vi "Main_E727_MultichannelMove.vi"() -> ()   [LabVIEW 2022 SP3]
doc: "This VI demonstrates how to initialize an E-727 system, how to move one connected axis and how to query for the position value of this axis. \nIn this example the E-727 is connected through COM port 1 with baudrate 115200. The VI runs E727_Configuration_Setup.vi with these specified settings, moves the first connected axis relative to its current position and reads the position of this axis. The diagram shows how to combine the driver VIs for these tasks. \nWarning: Before running this VI, modify the \"Interface\" and \"RS232 settings\" (or TCP/IP settings or USB settings ) to reflect your configuration. The predefined settings provided with the VI probably do not match your system."
uses:
  C:/Users/101d/Documents/Princeton Instruments/LightField/Add-in and Automation SDK/Samples/LabVIEW Automation/lightfield-automation-labview/LightField Automation.lvclass
panel:
  in  "Experiment Name:":u16(ring) items=["600IRWide", "1200SiWide"]
  in  "Tab Control":enum32{"Referenced Move", "Non referenced move"}(tab)
  in  "Set Point 1":bool
  out "Point 1":dbl[](array[numeric])=[137.9507141, 145.0551147, 152.0245361] format="%.6f"
  out "Point 2":dbl[](array[numeric])=[138.5597992, 116.5416107, 151.9612579] format="%.6f"
  in  "Set Point 2":bool
  in  "Start Mapping":bool
  out "Starting location":dbl[](array[numeric])=[136.47789, 224.1664276, 151.9103088] format="%.6f"
  in  "Set Starting location":bool
  in  "Left(-)/Right(+)":bool=TRUE
  in  "Up(-)/Down(+)":bool=TRUE
  in  "Move to Point 1":bool
  in  "Move to Point 2":bool
  in  "Move to \nStarting location":bool
  out "Y Move history":dbl[](array[numeric])
  out "X Move history":dbl[](array[numeric])
  out "Corrected angle":dbl
  out "Abs y":dbl
  out "Abs x":dbl
  out "y point":dbl
  out "x point":dbl
  in  "Array distance, D (um)":dbl=28.51
  in  "Pitch (um)":dbl=4.8
  in  "NxN array size":i32
  out "Inital position":dbl[](array[numeric]) format="%.6f"
  in  "Relative Resolution (um)":dbl[](array[numeric]) format="%.6f"
  in  "Map size":i32=7
  in  "Type of Motion":bool=TRUE
  in  "Target AbsolutePosition (um)":dbl[](array[numeric])=[150.0, 150.0, 150.0] format="%.6f"
  out "StageRunning 2":bool
  out "StageRunning 3":bool
  in  "Start Move":bool
  in  "Shut down":bool
  out "Position":dbl[](array[numeric]) format="%.6f"
  out "StageChannels":string[](array[string])
  in  "X / Y Resolution (um)":dbl=1.0 min=1.0
  in  "Z Resolution (um)":dbl=1.0 min=1.0
  in  "Left x0.5":bool
  in  "Right x0.5":bool
  in  "Up x0.5":bool
  in  "Down x0.5":bool
  in  "Down Z x4":bool
  in  "Down Z x2":bool
  in  "Up Z x4":bool
  in  "Up Z x2":bool
  in  "Up Z":bool
  in  "Down Z":bool
  in  "Right x4":bool
  in  "Right x2":bool
  in  "Left x4":bool
  in  "Left x2":bool
  in  "Down x4":bool
  in  "Down x2":bool
  in  "Up x4":bool
  in  "Up x2":bool
  in  "Right":bool
  in  "Left":bool
  in  "Up":bool
  in  "Down":bool
  out "LFRunning":bool
  out "LFObject":refnum<class "LightField Automation.lvclass">
  in  "LightFieldOn/Off":bool
  out "Progress":dbl(slide) scale=0.0..100.0
  out "Loop counter":dbl
  in  "error in":errorcluster
  out "StageRunning":bool
  in  "StageOn/Off":bool
  out "Pre-move position":dbl[](array[numeric]) format="%.6f"
  in  "stop":bool
  out "error out":errorcluster
  out "Current position":dbl[](array[numeric]) format="%.6f"
  # "Free relative move"
  # "Z Focus"
  # "X / Y Navigation"
  # "Lightfield"
  # "Y\nX\nZ"
  # "Flick to the direction of scan you want.\ne.g. default will move mapping right and up.\ngoing from bottom left to top right"
  # "Relative mapping\nRequires lightfield to be \"on\"\nThis will perform scans based on relative position and move in an \"S\" shape\nRelative solution is the length the stage will move per scan both in the X and Y axis\nMap size is the NxN scans it will take"
  # "Relative motion"
  # "Absolute motion"
  # "Relative Mapping settings"
  # "Y"
  # "X"
  # "Relative moving path"
  # "Z"
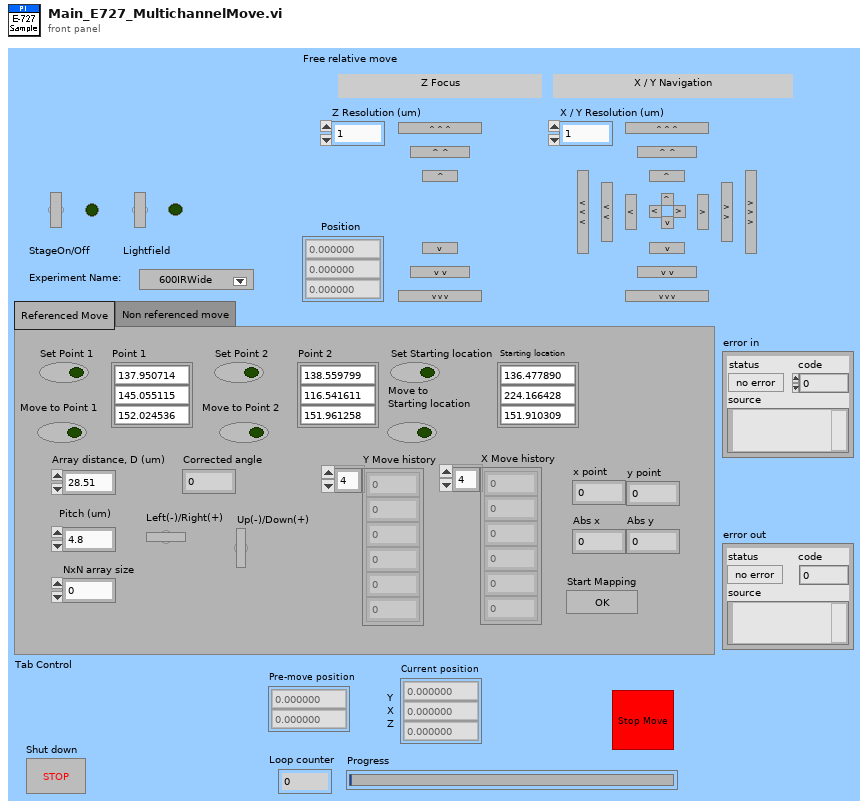
[diagram p1: front panel]
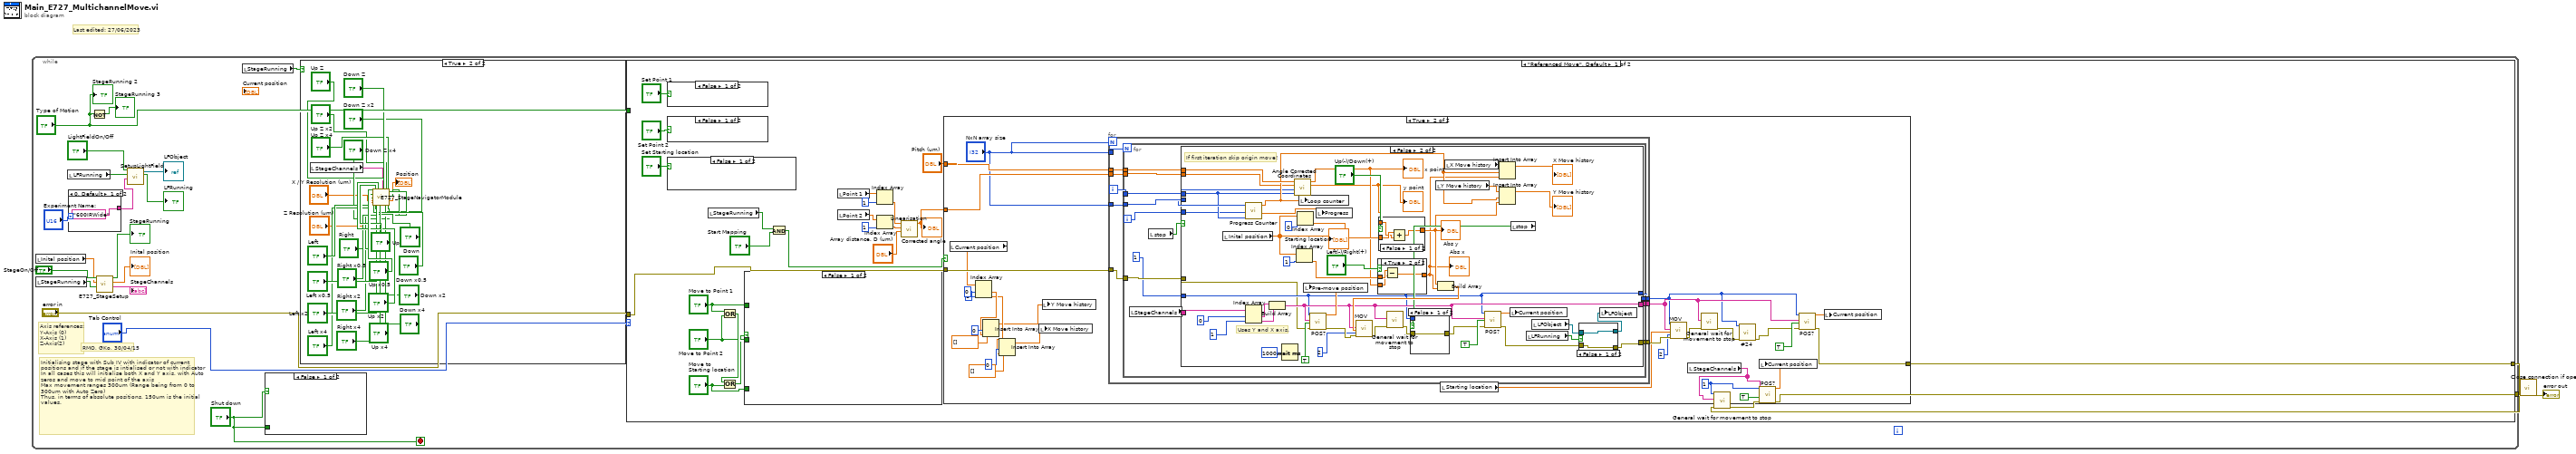
[diagram p0: block diagram]
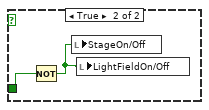
[diagram p2: hidden frame]
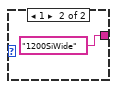
[diagram p3: hidden frame]
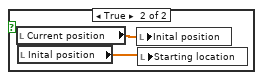
[diagram p4: hidden frame]
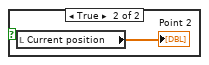
[diagram p5: hidden frame]
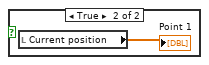
[diagram p6: hidden frame]
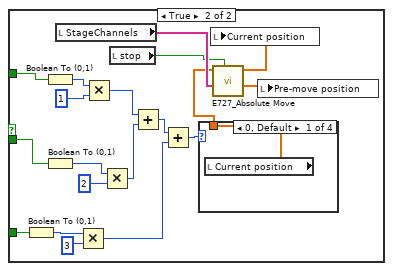
[diagram p7: hidden frame]
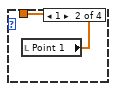
[diagram p8: hidden frame]
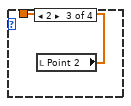
[diagram p9: hidden frame]
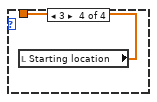
[diagram p10: hidden frame]
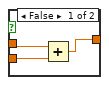
[diagram p13: hidden frame]
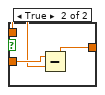
[diagram p14: hidden frame]
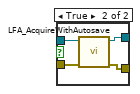
[diagram p15: hidden frame]
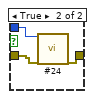
[diagram p16: hidden frame]
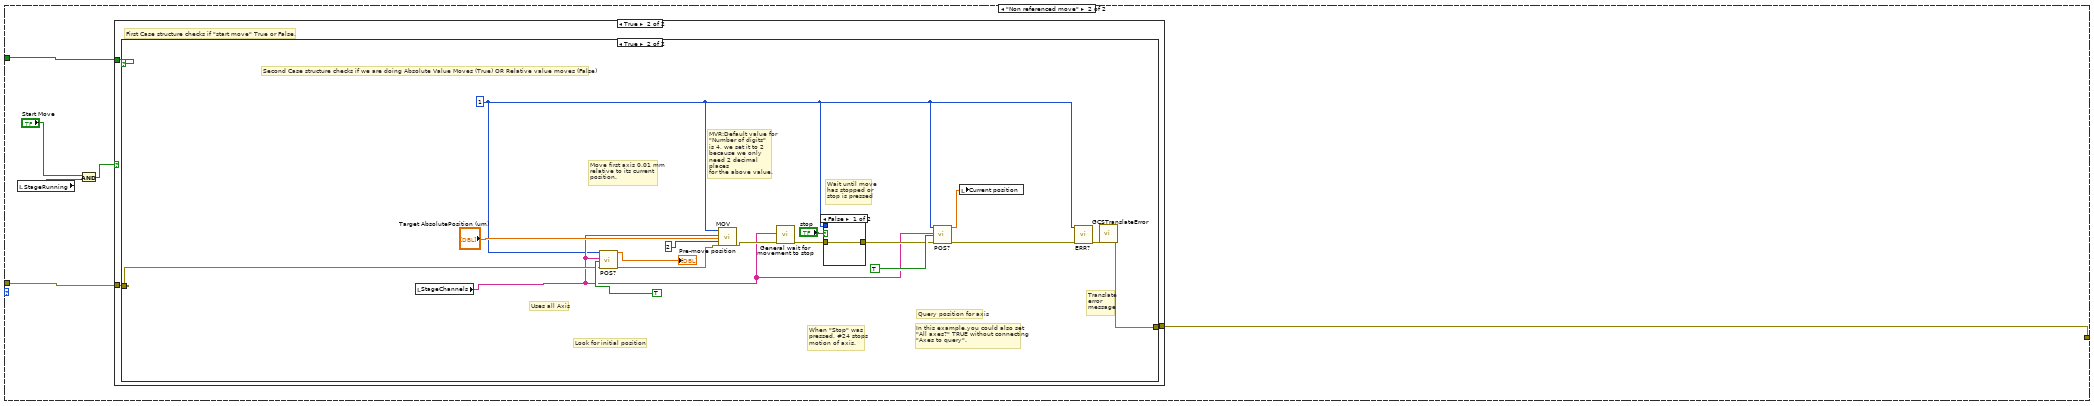
[diagram p17: hidden frame]
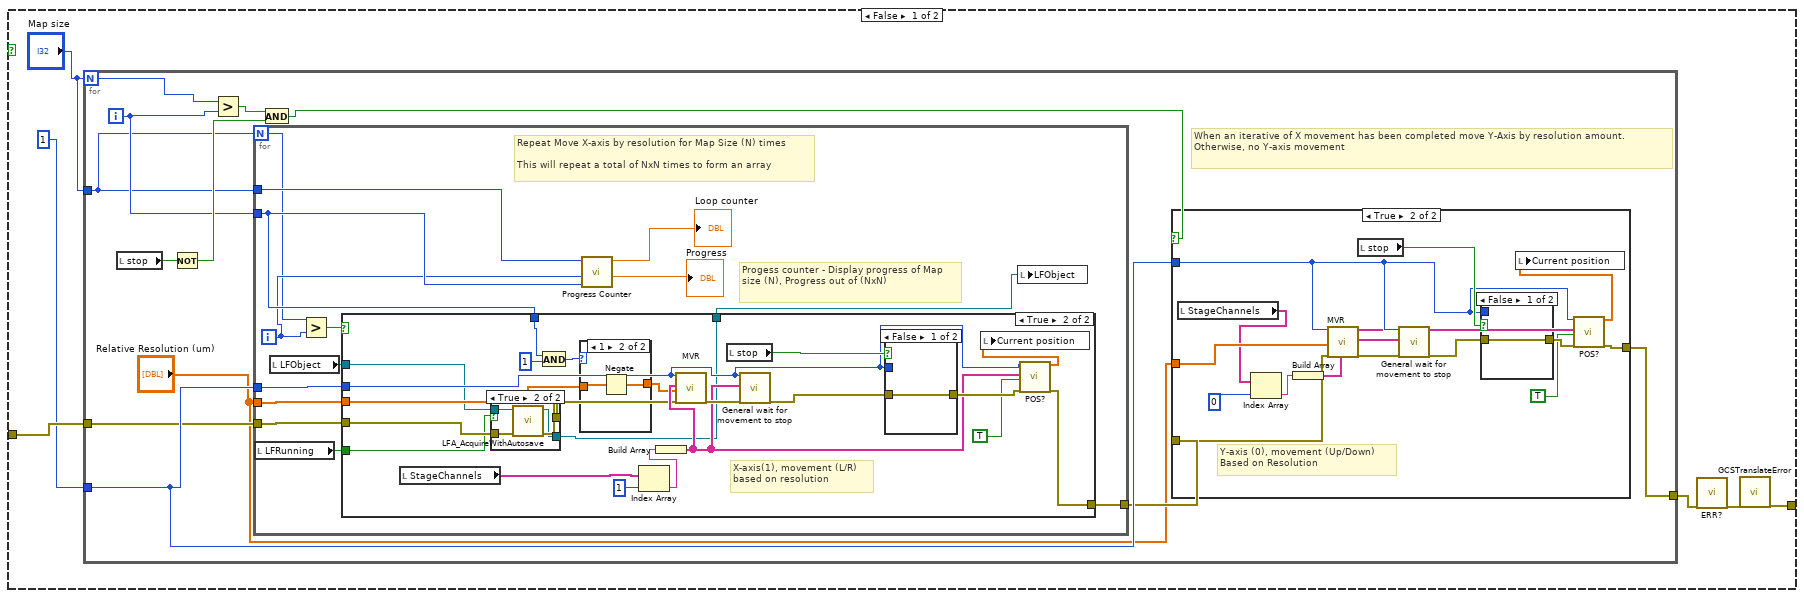
[diagram p19: hidden frame]
diagram:
  # "Last edited: 27/06/2023"
  n1 = while {
    tunnel: [w16] -> w1
    stop <- "Shut down" stop-if-true
    w12 = 1 ("System no.")
    # "Axis references:\nY-Axis (0)\nX-Axis (1)\nZ-Axis(2)"
    # "Initialising stage with Sub IV with indicator of current positions and if the stage is intialised or not with indicator\nIn all cases this will initialise both X and Y axis, with Auto zeros and move to mid point of the axis \nMax movement ranges 300um (Range being from 0 to 300um with Auto Zero)\nThus, in terms of absolute positions, 150um is the initial values."
    # "RMO, GKo, 30/04/15"
    n2 = local read "Inital position"() -> (w19:dbl[])
    n3 = local read "StageRunning"() -> (w6:bool)
    n4 = local read "LFRunning"() -> (w22:bool)
    n5 = case shown="0, Default" "Experiment Name:" {
      tunnel: ["600IRWide" "1200SiWide"] -> w4
      frame 0, Default {
      }
      frame 1 {
      }
    }
    n6 = Not(x="Type of Motion") -> (.not. x?=→"StageRunning 3":bool)
    n7 = call "E727_StageSetup.vi"("StageRunningIn"=w6, "Position 2"=w19, "StageOn/Off"="StageOn/Off") -> ("StageChannels"=→"StageChannels":string[], "Current position"=→"Inital position":dbl[], "StageRunningOut"=→"StageRunning":bool)  [unwired: 5 in, 1 out]
    n8 = call "SetupLightField.vi"("Experiment Name:"=w4, "LFRunningIn"=w22, "LFOn/Off"="LightFieldOn/Off") -> ("LFRunning"=→"LFRunning":bool, "LFObject"=→"LFObject":refnum<class "LightField Automation.lvclass">)  [unwired: 7 in]
    n9 = local read "StageRunning"() -> (w18:bool)
    n10 = case shown="False" "Shut down" {
      tunnel: "Shut down" -> [_ w29]
      frame False {
      }
      frame True {
        n11 = Not(x=w29) -> (.not. x?=w28:bool)
        n12 = local write "StageOn/Off"(w28) -> ()
        n13 = local write "LightFieldOn/Off"(w28) -> ()
      }
    }
    n14 = case shown="True" w18 {
      frame False {
      }
      frame True {
        n15 = local read "StageChannels"() -> (w321:string[])
        n16 = call "E727_StageNavigatorModule.vi"("Up Z x4"="Up Z x4", "Up Z x2"="Up Z x2", "Up Z"="Up Z", "StageChannels"=w321, "Up x4"="Up x4", "Up x2"="Up x2", "Up"="Up", "Up x0.5"="Up x0.5", "Right x0.5"="Right x0.5", "Left x0.5"="Left x0.5", "Right"="Right", "Left"="Left", "Right x2"="Right x2", "Left x2"="Left x2", "Right x4"="Right x4", "Left x4"="Left x4", "X / Y Resolution (um)"="X / Y Resolution (um)", "Z Resolution (um)"="Z Resolution (um)", "Down Z x4"="Down Z x4", "Down Z x2"="Down Z x2", "Down Z"="Down Z", "Down x4"="Down x4", "Down x2"="Down x2", "Down"="Down", "Down x0.5"="Down x0.5") -> ("Position"=→"Position":dbl[])  [unwired: 2 in]
      }
    }
    n17 = case shown="\"Referenced Move\", Default" "Tab Control" {
      tunnel: "error in" -> [w32 w206]
      tunnel: "Type of Motion" -> [_ w205]
      tunnel: [w33 w204] -> w7
      frame "Referenced Move", Default {
        n18 = case shown="False" "Set Point 1" {
          frame False {
          }
          frame True {
            n19 = local read "Current position"() -> (→"Point 1":dbl[])
          }
        }
        n20 = case shown="False" "Set Point 2" {
          frame False {
          }
          frame True {
            n21 = local read "Current position"() -> (→"Point 2":dbl[])
          }
        }
        n22 = case shown="False" "Set Starting location" {
          frame False {
          }
          frame True {
            n23 = local read "Current position"() -> (w55:dbl[])
            n24 = local read "Inital position"() -> (w54:dbl[])
            n25 = local write "Inital position"(w55) -> ()
            n26 = local write "Starting location"(w54) -> ()
          }
        }
        n27 = local read "StageRunning"() -> (w36:bool)
        n28 = Or(x="Move to Point 1", y="Move to Point 2") -> (x .or. y?=w44:bool)
        n29 = Or(x=w44, y="Move to \nStarting location") -> (x .or. y?=w40:bool)
        n30 = case shown="False" w40 {
          tunnel: "Move to Point 1" -> [_ w76]
          tunnel: "Move to Point 2" -> [_ w75]
          tunnel: "Move to \nStarting location" -> [_ w74]
          frame False {
          }
          frame True {
            n31 = Boolean To (0,1)(Boolean=w74) -> (0, 1=w69:i16)
            n32 = Boolean To (0,1)(Boolean=w76) -> (0, 1=w73:i16)
            n33 = Boolean To (0,1)(Boolean=w75) -> (0, 1=w71:i16)
            n34 = local read "StageChannels"() -> (w62:string[])
            n35 = Multiply(x=w69, y=i16 3) -> (x*y=w65:i16)
            n36 = Multiply(x=w73, y=i16 1) -> (x*y=w67:i16)
            n37 = Multiply(x=w71, y=i16 2) -> (x*y=w66:i16)
            n38 = local read "stop"() -> (w58:bool)
            n39 = Add(x=w67, y=w66) -> (x+y=w64:i16)
            n40 = Add(x=w64, y=w65) -> (x+y=w63:i16)
            n41 = case shown="0, Default" w63 {
              tunnel: [w77 w78 w79 w80] -> w61
              frame 0, Default {
                n42 = local read "Current position"() -> (w77:dbl[])
              }
              frame 1 {
                n43 = local read "Point 1"() -> (w78:dbl[])
              }
              frame 2 {
                n44 = local read "Point 2"() -> (w79:dbl[])
              }
              frame 3 {
                n45 = local read "Starting location"() -> (w80:dbl[])
              }
            }
            n46 = call "E727_Absolute Move.vi"("Target AbsolutePosition (um)"=w61, "StageChannels 2"=w62, "stop 2"=w58) -> ("Current position"=w60:dbl[], "Pre-move position 2"=w59:dbl[])  [unwired: 6 in]
            n47 = local write "Current position"(w60) -> ()
            n48 = local write "Pre-move position"(w59) -> ()
          }
        }
        n49 = And(x=w36, y="Start Mapping") -> (x .and. y?=w34:bool)
        n50 = local read "Point 1"() -> (w51:dbl[])
        n51 = local read "Point 2"() -> (w50:dbl[])
        n52 = Index Array(array=w51, index=1) -> (element=w52:dbl)
        n53 = Index Array(array=w50, index=1) -> (element=w53:dbl)
        n54 = call "Linearisation.vi"("Array distance, D (um)"="Array distance, D (um)", "x point 2"=w53, "x point 1"=w52) -> ("Corrected angle"=w48:dbl)  [unwired: 8 in]
        "Corrected angle" <- w48
        n55 = case shown="True" w34 {
          tunnel: "Pitch (um)" -> [_ w107]
          tunnel: w48 -> [_ w106]
          tunnel: [w81 w94] -> w33
          tunnel: w32 -> [w81 w93]
          frame False {
          }
          frame True {
            n56 = local read "Current position"() -> (w92:dbl[])
            n57 = Index Array(array=w92, index #1=0 ("index"), index #2=1 ("index")) -> (element #1=w87:dbl, element #2=w86:dbl)
            n58 = Insert Into Array(array=dbl[] [], index=0, new element=w87) -> (w84:dbl[])
            n59 = Insert Into Array(array=dbl[] [], index=0, new element=w86) -> (w85:dbl[])
            n60 = local write "X Move history"(w85) -> ()
            n61 = local write "Y Move history"(w84) -> ()
            n62 = for {
              N: "NxN array size" -> [_]
              tunnel: w107 -> [w116]
              tunnel: w106 -> [w115]
              tunnel: "NxN array size" -> [w114]
              tunnel: "NxN array size" -> [w113]
              tunnel: [w112] -> w102
              tunnel: [w111] -> w97
              tunnel: [w110] -> w98
              tunnel: w93 -> [w109]
              i -> [w108]
              n63 = for {
                N: w114 -> [_]
                tunnel: w116 -> [w128]
                tunnel: w115 -> [w127]
                tunnel: w108 -> [w125]
                tunnel: w113 -> [w124]
                tunnel: [w123] -> w112
                tunnel: [w119] -> w111
                tunnel: w109 -> [w122]
                tunnel: [w121] -> w110
                i -> [w126]
                n64 = local read "StageChannels"() -> (w118:string[])
                n65 = local read "stop"() -> (w117:bool)
                n66 = case shown="False" w117 {
                  tunnel: w128 -> [_ w178]
                  tunnel: w127 -> [_ w136]
                  tunnel: w126 -> [_ w135]
                  tunnel: w125 -> [_ w140]
                  tunnel: w124 -> [_ w158]
                  tunnel: [w130 w138] -> w123
                  tunnel: w122 -> [w130 w137]
                  tunnel: [w129 w151] -> w121
                  tunnel: 1 ("System no.") -> [w131 w150]
                  tunnel: [w131 w150] -> w119
                  tunnel: w118 -> [w129 w149]
                  frame True {
                  }
                  frame False {
                    # "If first iteration skip origin move!"
                    # "Uses Y and X axis."
                    n67 = local read "Inital position"() -> (w162:dbl[])
                    "Starting location" <- w162
                    n68 = Index Array(array=w149, index #1=0 ("index"), index #2=1 ("index")) -> (element #1=w170:string, element #2=w165:string)
                    n69 = call "Progress Counter.vi"("y"=w140, "x"=w135, "Map size (Pixels)"=w158) -> ("Progress"=w157:dbl, "Loop counter"=w141:dbl)  [unwired: 7 in]
                    n70 = Build Array(w170, w165) -> (w151:string[])
                    n71 = Wait (ms)(milliseconds to wait=u32 1000) -> ()  [unwired: 1 out]
                    n72 = call "Angle Corrected Coordinates.vi"("Outer iteration"=w140, "Inner iteration"=w135, "Corrected angle"=w136, "Pitch (um)"=w178) -> ("y position"=w134:dbl, "x position"=w146:dbl)  [unwired: 1 in, 1 out]
                    "x point" <- w146
                    "y point" <- w134
                    n73 = Index Array(array=w162, index=1) -> (element=w153:dbl)
                    n74 = Index Array(array=w162, index=0) -> (element=w152:dbl)
                    n75 = local write "Loop counter"(w141) -> ()
                    n76 = call "POS?.vi"("System no."=w150, "Axes to query"=w151, "All axes?"=TRUE, "error in"=w137) -> ("Position"=w163:dbl[], "error out"=w168:errorcluster)  [unwired: 1 in, 13 out]
                    n77 = local write "Pre-move position"(w163) -> ()
                    n78 = local write "Progress"(w157) -> ()
                    n79 = case shown="True" "Left(-)/Right(+)" {
                      tunnel: w153 -> [w181 w184]
                      tunnel: [w179 w183] -> w132
                      tunnel: w146 -> [w180 w182]
                      frame False {
                        n80 = Add(x=w181, y=w180) -> (x+y=w179:dbl)
                      }
                      frame True {
                        n81 = Subtract(x=w184, y=w182) -> (x-y=w183:dbl)
                      }
                    }
                    "Abs x" <- w132
                    n82 = case shown="False" "Up(-)/Down(+)" {
                      tunnel: w152 -> [w187 w190]
                      tunnel: [w185 w189] -> w133
                      tunnel: w134 -> [w186 w188]
                      frame False {
                        n83 = Add(x=w187, y=w186) -> (x+y=w185:dbl)
                      }
                      frame True {
                        n84 = Subtract(x=w190, y=w188) -> (x-y=w189:dbl)
                      }
                    }
                    "Abs y" <- w133
                    n85 = local read "Y Move history"() -> (w142:dbl[])
                    n86 = Build Array(w133, w132) -> (w161:dbl[])
                    n87 = call "MOV.vi"("Axes to move"=w151, "Position values"=w161, "No.of digits"=i16 2, "error in"=w168) -> ("error out"=w167:errorcluster)  [unwired: 1 in, 14 out]
                    n88 = call "General wait for movement to stop.vi"("Axes to wait for"=w151, "error in"=w167) -> ("error out"=w173:errorcluster)  [unwired: 6 in, 11 out]
                    n89 = local read "X Move history"() -> (w143:dbl[])
                    n90 = Insert Into Array(array=w143, index=w141, new element=w132) -> (→"X Move history":dbl[])
                    n91 = Insert Into Array(array=w142, index=w141, new element=w133) -> (→"Y Move history":dbl[])
                    n92 = local read "stop"() -> (w159:bool)
                    n93 = case shown="False" w159 {
                      tunnel: w173 -> [w197 w200]
                      tunnel: [w197 w199] -> w172
                      tunnel: w150 -> [_ w198]
                      frame False {
                      }
                      frame True {
                        n94 = call "#24.vi"("System no."=w198, "error in"=w200) -> ("error out"=w199:errorcluster)  [unwired: 17 out]
                      }
                    }
                    n95 = call "POS?.vi"("System no."=w150, "Axes to query"=w151, "All axes?"=TRUE, "error in"=w172) -> ("Position"=w160:dbl[], "error out"=w139:errorcluster)  [unwired: 1 in, 13 out]
                    n96 = local write "Current position"(w160) -> ()
                    n97 = local read "LFRunning"() -> (w154:bool)
                    n98 = local read "LFObject"() -> (w156:refnum<class "LightField Automation.lvclass">)
                    n99 = case shown="False" w154 {
                      tunnel: w139 -> [w192 w196]
                      tunnel: [w192 w195] -> w138
                      tunnel: [w191 w194] -> w155
                      tunnel: w156 -> [w191 w193]
                      frame False {
                      }
                      frame True {
                        n100 = call "LFA_AcquireWithAutosave.vi"("error in (no error)"=w196, "LightField Automation in"=w193) -> ("error out"=w195:errorcluster, "LightField Automation out"=w194:refnum<class "LightField Automation.lvclass">)  [unwired: 7 in, 1 out]
                      }
                    }
                    n101 = local write "LFObject"(w155) -> ()
                  }
                }
              }
            }
            n102 = local read "Starting location"() -> (w96:dbl[])
            n103 = call "MOV.vi"("System no."=w97, "Axes to move"=w98, "Position values"=w96, "No.of digits"=i16 2, "error in"=w102) -> ("error out"=w104:errorcluster)  [unwired: 14 out]
            n104 = call "General wait for movement to stop.vi"("Axes to wait for"=w98, "error in"=w104) -> ("error out"=w101:errorcluster)  [unwired: 6 in, 11 out]
            n105 = call "#24.vi"("System no."=w97, "error in"=w101) -> ("error out"=w100:errorcluster)  [unwired: 17 out]
            n106 = call "POS?.vi"("System no."=w97, "Axes to query"=w98, "All axes?"=TRUE, "error in"=w100) -> ("Position"=w105:dbl[], "error out"=w94:errorcluster)  [unwired: 1 in, 13 out]
            n107 = local write "Current position"(w105) -> ()
          }
        }
      }
      frame "Non referenced move" {
        n108 = local read "StageRunning"() -> (w201:bool)
        n109 = And(x="Start Move", y=w201) -> (x .and. y?=w203:bool)
        n110 = case shown="True" w203 {
          tunnel: w206 -> [w207 w209]
          tunnel: [w207 w210] -> w204
          tunnel: w205 -> [_ w208]
          frame False {
          }
          frame True {
            # "First Case structure checks if \"start move\" True or False,"
            n111 = case shown="True" w208 {
              tunnel: [w213 w308] -> w210
              tunnel: w209 -> [w214 w306]
              frame False {
                n112 = for {
                  N: "Map size" -> [w219]
                  tunnel: "Map size" -> [w217]
                  tunnel: w214 -> [w225]
                  tunnel: 1 ("System no.") -> [w226]
                  tunnel: [w222] -> w212
                  i -> [w220]
                  # "When an iterative of X movement has been completed move Y-Axis by resolution amount.\nOtherwise, no Y-axis movement"
                  n113 = local read "stop"() -> (w227:bool)
                  n114 = Not(x=w227) -> (.not. x?=w228:bool)
                  n115 = Greater?(x=w219, y=w220) -> (0:w221:bool)
                  n116 = for {
                    N: w217 -> [w252]
                    tunnel: w225 -> [w261]
                    tunnel: w226 -> [w260]
                    tunnel: "Relative Resolution (um)" -> [w259]
                    tunnel: w217 -> [w258]
                    tunnel: w220 -> [w255]
                    tunnel: [w256] -> w223
                    i -> [w254]
                    # "Repeat Move X-axis by resolution for Map Size (N) times\n\nThis will repeat a total of NxN times to form an array"
                    # "Progess counter - Display progress of Map size (N), Progress out of (NxN)"
                    n117 = local read "LFRunning"() -> (w249:bool)
                    n118 = local read "LFObject"() -> (w250:refnum<class "LightField Automation.lvclass">)
                    n119 = Greater?(x=w252, y=w254) -> (0:w253:bool)
                    n120 = case shown="True" w253 {
                      tunnel: w261 -> [w263 w269]
                      tunnel: w260 -> [_ w279]
                      tunnel: w259 -> [_ w271]
                      tunnel: [w263 w277] -> w256
                      tunnel: w255 -> [_ w273]
                      tunnel: [w262 w267] -> w251
                      tunnel: w250 -> [w262 w266]
                      tunnel: w249 -> [_ w265]
                      frame False {
                      }
                      frame True {
                        # "X-axis(1), movement (L/R) based on resolution"
                        n121 = local read "StageChannels"() -> (w264:string[])
                        n122 = case shown="True" w265 {
                          tunnel: w269 -> [w287 w291]
                          tunnel: [w287 w290] -> w268
                          tunnel: [w286 w289] -> w267
                          tunnel: w266 -> [w286 w288]
                          frame False {
                          }
                          frame True {
                            n123 = call "LFA_AcquireWithAutosave.vi"("error in (no error)"=w291, "LightField Automation in"=w288) -> ("error out"=w290:errorcluster, "LightField Automation out"=w289:refnum<class "LightField Automation.lvclass">)  [unwired: 7 in, 1 out]
                          }
                        }
                        n124 = And(x=w273, y=1) -> (x .and. y?=w275:i32)
                        n125 = case shown="1" w275 {
                          tunnel: [w292 w293] -> w272
                          tunnel: w271 -> [w292 w294]
                          frame 0, Default {
                          }
                          frame 1 {
                            n126 = Negate(x=w294) -> (-x=w293:dbl[])
                          }
                        }
                        n127 = Index Array(array=w264, index=1) -> (element=w283:string)
                        n128 = Build Array(w283) -> (w278:string[])
                        n129 = call "MVR.vi"("System no."=w279, "Axes to move"=w278, "Position values"=w272, "error in"=w268) -> ("error out"=w285:errorcluster)  [unwired: 1 in, 14 out]
                        n130 = local read "stop"() -> (w280:bool)
                        n131 = call "General wait for movement to stop.vi"("System no."=w279, "Axes to wait for"=w278, "error in"=w285) -> ("error out"=w282:errorcluster)  [unwired: 5 in, 11 out]
                        n132 = case shown="False" w280 {
                          tunnel: w282 -> [w295 w298]
                          tunnel: [w295 w297] -> w281
                          tunnel: w279 -> [_ w296]
                          frame False {
                          }
                          frame True {
                            n133 = call "#24.vi"("System no."=w296, "error in"=w298) -> ("error out"=w297:errorcluster)  [unwired: 17 out]
                          }
                        }
                        n134 = call "POS?.vi"("System no."=w279, "Axes to query"=w278, "All axes?"=TRUE, "error in"=w281) -> ("Position"=w276:dbl[], "error out"=w277:errorcluster)  [unwired: 1 in, 13 out]
                        n135 = local write "Current position"(w276) -> ()
                      }
                    }
                    n136 = call "Progress Counter.vi"("y"=w255, "x"=w254, "Map size (Pixels)"=w258) -> ("Progress"=→"Progress":dbl, "Loop counter"=→"Loop counter":dbl)  [unwired: 7 in]
                    n137 = local write "LFObject"(w251) -> ()
                  }
                  n138 = And(x=w221, y=w228) -> (x .and. y?=w224:bool)
                  n139 = case shown="True" w224 {
                    tunnel: w226 -> [_ w233]
                    tunnel: w223 -> [w229 w240]
                    tunnel: "Relative Resolution (um)" -> [_ w237]
                    tunnel: [w229 w235] -> w222
                    frame False {
                    }
                    frame True {
                      # "Y-axis (0), movement (Up/Down)\nBased on Resolution"
                      n140 = local read "StageChannels"() -> (w230:string[])
                      n141 = Index Array(array=w230, index=0) -> (element=w242:string)
                      n142 = Build Array(w242) -> (w232:string[])
                      n143 = call "MVR.vi"("System no."=w233, "Axes to move"=w232, "Position values"=w237, "error in"=w240) -> ("error out"=w241:errorcluster)  [unwired: 1 in, 14 out]
                      n144 = local read "stop"() -> (w239:bool)
                      n145 = call "General wait for movement to stop.vi"("System no."=w233, "Axes to wait for"=w232, "error in"=w241) -> ("error out"=w238:errorcluster)  [unwired: 5 in, 11 out]
                      n146 = case shown="False" w239 {
                        tunnel: w238 -> [w244 w247]
                        tunnel: [w244 w246] -> w236
                        tunnel: w233 -> [_ w245]
                        frame False {
                        }
                        frame True {
                          n147 = call "#24.vi"("System no."=w245, "error in"=w247) -> ("error out"=w246:errorcluster)  [unwired: 17 out]
                        }
                      }
                      n148 = call "POS?.vi"("System no."=w233, "Axes to query"=w232, "All axes?"=TRUE, "error in"=w236) -> ("Position"=w234:dbl[], "error out"=w235:errorcluster)  [unwired: 1 in, 13 out]
                      n149 = local write "Current position"(w234) -> ()
                    }
                  }
                }
                n150 = call "ERR?.vi"("error in"=w212) -> ("error out"=w215:errorcluster)  [unwired: 1 in, 17 out]
                n151 = call "GCSTranslateError.vi"("error in"=w215) -> ("error out"=w213:errorcluster)  [unwired: 18 out]
              }
              frame True {
                w299 = 1 ("System no.")
                # "Look for initial position"
                # "Second Case structure checks if we are doing Absolute Value Moves (True) OR Relative value moves (False)"
                # "Uses all Axis"
                # "When \"Stop\" was \npressed, #24 stops\nmotion of axis."
                # "Translate\nerror \nmessage"
                # "Wait until move\nhas stopped or\nstop is pressed"
                # "MVR:Default value for\n\"Number of digits\"\nis 4, we set it to 2\nbecause we only\nneed 2 decimal places\nfor the above value."
                # "Move first axis 0.01 mm\nrelative to its current\nposition."
                # "In this example,you could also set \n\"All axes?\" TRUE without connecting\n\"Axes to query\"."
                # "Query position for axis"
                n152 = local read "StageChannels"() -> (w300:string[])
                n153 = call "POS?.vi"("System no."=w299, "Axes to query"=w300, "All axes?"=TRUE, "error in"=w306) -> ("Position"=→"Pre-move position":dbl[], "error out"=w305:errorcluster)  [unwired: 1 in, 13 out]
                n154 = call "MOV.vi"("System no."=w299, "Axes to move"=w300, "Position values"="Target AbsolutePosition (um)", "No.of digits"=i16 2, "error in"=w305) -> ("error out"=w304:errorcluster)  [unwired: 14 out]
                n155 = call "General wait for movement to stop.vi"("Axes to wait for"=w300, "error in"=w304) -> ("error out"=w314:errorcluster)  [unwired: 6 in, 11 out]
                n156 = case shown="False" "stop" {
                  tunnel: w314 -> [w316 w319]
                  tunnel: [w316 w318] -> w313
                  tunnel: w299 -> [_ w317]
                  frame False {
                  }
                  frame True {
                    n157 = call "#24.vi"("System no."=w317, "error in"=w319) -> ("error out"=w318:errorcluster)  [unwired: 17 out]
                  }
                }
                n158 = call "POS?.vi"("System no."=w299, "Axes to query"=w300, "All axes?"=TRUE, "error in"=w313) -> ("Position"=w301:dbl[], "error out"=w311:errorcluster)  [unwired: 1 in, 13 out]
                n159 = local write "Current position"(w301) -> ()
                n160 = call "ERR?.vi"("System no."=w299, "error in"=w311) -> ("error out"=w310:errorcluster)  [unwired: 17 out]
                n161 = call "GCSTranslateError.vi"("error in"=w310) -> ("error out"=w308:errorcluster)  [unwired: 18 out]
              }
            }
          }
        }
      }
    }
    n162 = local read "StageChannels"() -> (w11:string[])
    n163 = call "General wait for movement to stop.vi"("System no."=w12, "Axes to wait for"=w11, "error in"=w7) -> ("error out"=w13:errorcluster)  [unwired: 5 in, 11 out]
    n164 = call "POS?.vi"("System no."=w12, "Axes to query"=w11, "All axes?"=TRUE, "error in"=w13) -> ("Position"=w15:dbl[], "error out"=w16:errorcluster)  [unwired: 1 in, 13 out]
    n165 = local write "Current position"(w15) -> ()
    "StageRunning 2" <- "Type of Motion"
  }
  n166 = call "Close connection if open.vi"("error in"=w1) -> ("error out"=→"error out":errorcluster)  [unwired: 2 in, 16 out]
